vi "Splash Screen.vi"(8 "error in":errorcluster) -> (0 "error out":errorcluster)   [LabVIEW 2021, in "Panther Dashboard.lvlib"]
uses:
  Panther Dashboard.lvlib
panel:
  out "Title and version":string
  out "Progress":u16(slide) scale=-1.0..30.0
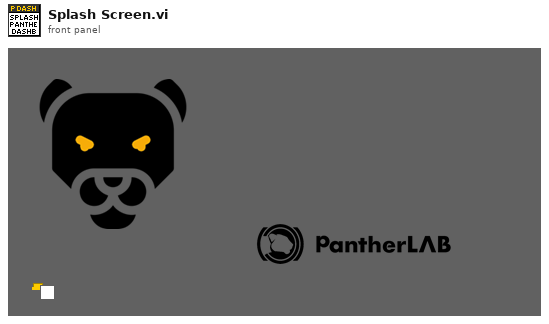
[diagram p1: front panel]
types:
  T1 = cluster{"Major":u16, "Minor":u16, "Fix":u16, "Build":u16}
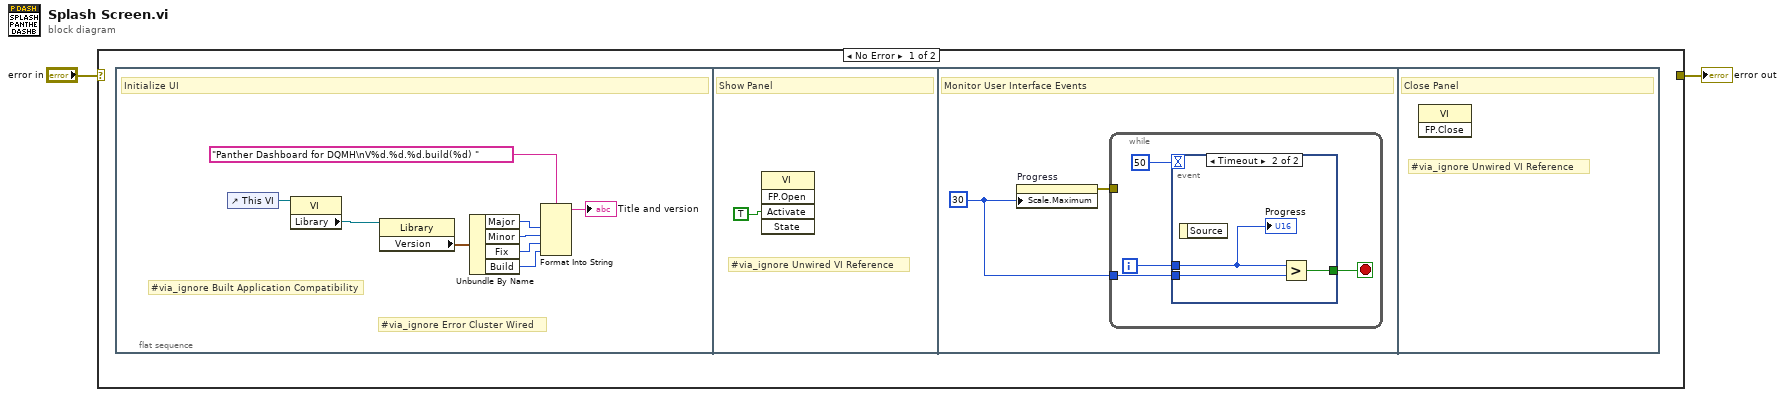
[diagram p0: block diagram]
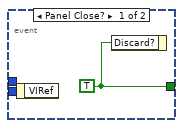
[diagram p2: hidden frame]
diagram:
  n1 = case shown="No Error" "error in" {
    selector: "error in" -> [_ w23]
    tunnel: [_ w23] -> w1
    frame No Error {
      n2 = flat-sequence {
        frame #0 {
          # "#via_ignore Built Application Compatibility"
          # "#via_ignore Error Cluster Wired"
          # "Initialize UI"
          n3 = control-ref of="This VI"() -> (w10:refnum<vi>)
          n4 = property class="VI"(reference=w10) -> ("Library"=w9:refnum<vi>)  [unwired: 1 in, 2 out]
          n5 = property class="Library"(reference=w9) -> ("Version"=w8:T1)  [unwired: 1 in, 2 out]
          n6 = Unbundle By Name(w8) -> ("Major"=w7:u16, "Minor"=w6:u16, "Fix"=w5:u16, "Build"=w4:u16)
          n7 = Format Into String(format string="Panther Dashboard for DQMH\nV%d.%d.%d.build(%d) " ("String"), w7, w6, w5, w4) -> (resulting string=→"Title and version":string)  [unwired: 2 in, 1 out]
        }
        frame #1 {
          # "#via_ignore Unwired VI Reference"
          # "Show Panel"
          n8 = invoke class="VI" method="FP.Open"("Activate"=TRUE ("Activate?")) -> ()  [unwired: 4 in, 5 out]
        }
        frame #2 {
          w13 = 30 ("y")
          # "Monitor User Interface Events"
          n9 = property on="Progress" class="Slide (strict)"("Scale.Maximum"=w13) -> (error out=w14:errorcluster)  [unwired: 2 in, 1 out]
          n10 = while {
            tunnel: w14 -> [_]
            tunnel: w13 -> [w15]
            i -> [w17]
            stop <- w18 stop-if-true
            n11 = event shown="[1] Timeout" {
              selector: _ -> [_ _]
              dyn-events: _ -> [_ _]
              timeout: 50 -> [_ _]
              tunnel: [w19 w22] -> w18
              tunnel: w17 -> [_ w21]
              tunnel: w15 -> [_ w20]
              event Panel Close? {
                w19 = TRUE ("Discard?")
                n12 = event-data() -> ()  [unwired: 1 in, 1 out]
                n13 = event-data("Discard?"=w19) -> ()  [unwired: 1 in, 1 out]
              }
              event Timeout {
                n14 = event-data() -> ()  [unwired: 1 in, 1 out]
                n15 = Greater?(x=w21, y=w20) -> (0:w22:bool)
                "Progress" <- w21
              }
            }
          }
        }
        frame #3 {
          # "#via_ignore Unwired VI Reference"
          # "Close Panel"
          n16 = invoke class="VI" method="FP.Close"() -> ()  [unwired: 3 in, 3 out]
        }
      }
    }
    frame Error {
    }
  }
  "error out" <- w1
